vi "test Basic Splitting of Elements.vi"(8 "error in (no error)":errorcluster, 11 "TestCase in":refnum<class "Package List Tests.lvclass">) -> (0 "error out":errorcluster, 3 "TestCase out":refnum<class "Package List Tests.lvclass">)   [LabVIEW 2015, in "Package List Tests.lvclass"]
uses:
  Package List Tests.lvclass
  <vilib>/addons/_JKI Toolkits/VI Tester/TestCase.llb/TestCase.lvclass
  G CLI VIP.lvlib
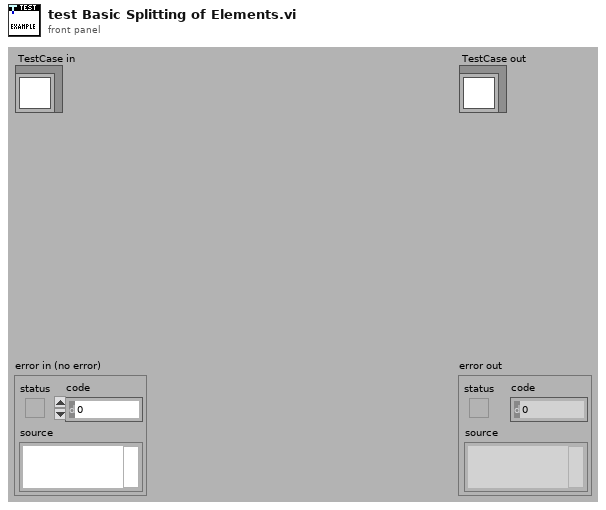
[diagram p1: front panel]
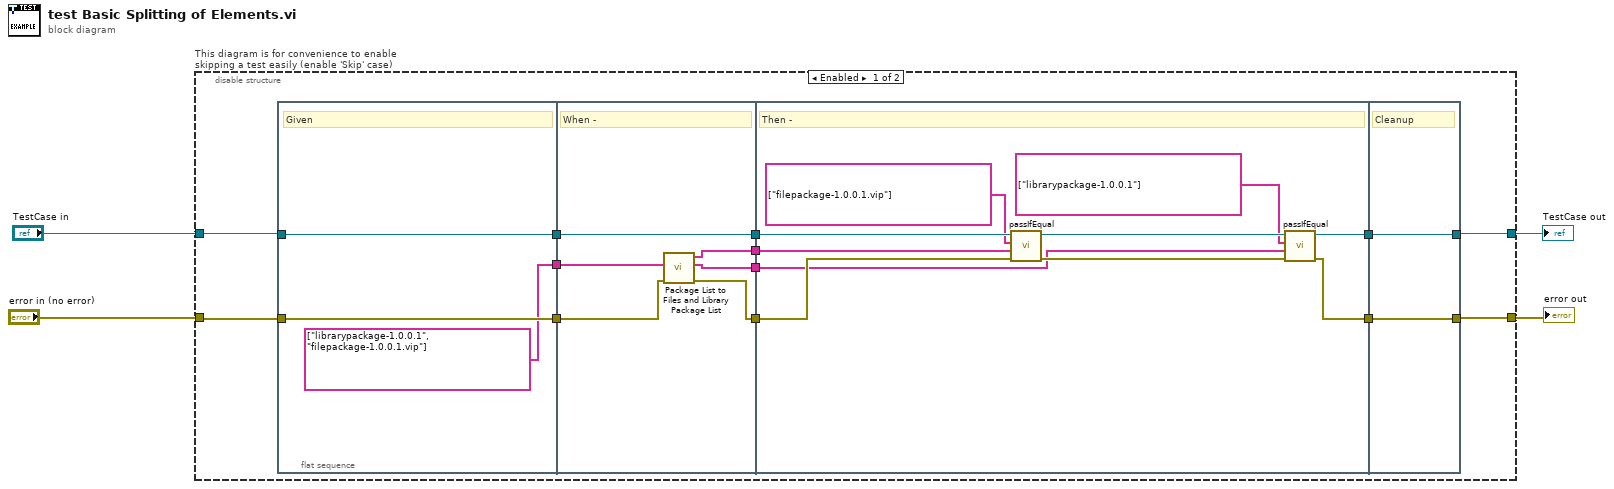
[diagram p0: block diagram]
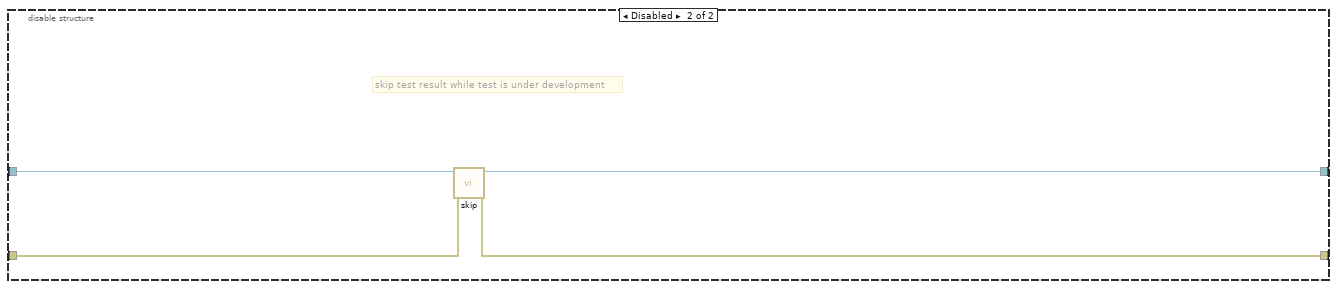
[diagram p2: hidden frame]
diagram:
  n1 = disable-structure "This diagram is for convenience to enable skipping a test easily (enable 'Skip' case)" shown="Enabled" {
    disable-tunnel: "TestCase in" -> [w12 w42]
    disable-tunnel: [w10 w40] -> w1
    disable-tunnel: [w9 w41] -> w3
    disable-tunnel: "error in (no error)" -> [w11 w39]
    frame Enabled {
      n2 = flat-sequence {
        tunnel: w11 -> [w19]
        tunnel: w12 -> [w20]
        tunnel: [w20] -> w17
        tunnel: [w19] -> w16
        tunnel: [string[] ["librarypackage-1.0.0.1", "filepackage-1.0.0.1.vip"]] -> w8
        tunnel: [w26] -> w15
        tunnel: w17 -> [w26]
        tunnel: w16 -> [w22]
        tunnel: w8 -> [w25]
        tunnel: [w24] -> w7
        tunnel: [w23] -> w6
        tunnel: [w21] -> w5
        tunnel: [w31] -> w14
        tunnel: [w32] -> w13
        tunnel: w15 -> [w36]
        tunnel: w7 -> [w30]
        tunnel: w6 -> [w29]
        tunnel: w5 -> [w35]
        tunnel: [w38] -> w9
        tunnel: [w37] -> w10
        tunnel: w14 -> [w37]
        tunnel: w13 -> [w38]
        frame #0 {
          # "Given"
        }
        frame #1 {
          # "When -"
          n3 = call "Package List to Files and Library Package List.vi"("error in (no error)"=w22, "Packages"=w25) -> ("error out"=w21:errorcluster, "Library Packages"=w23:string[], "File Packages"=w24:string[])  [unwired: 7 in]
        }
        frame #2 {
          # "Then -"
          n4 = call-dynamic "passIfEqual.vi"("error in (no error)"=w35, "y"=w30, "x"=string[] ["filepackage-1.0.0.1.vip"], "TestCase in"=w36) -> ("error out"=w33:errorcluster, "TestCase out"=w34:refnum<class "Package List Tests.lvclass">)  [unwired: 6 in]
          n5 = call-dynamic "passIfEqual.vi"("error in (no error)"=w33, "y"=w29, "x"=string[] ["librarypackage-1.0.0.1"], "TestCase in"=w34) -> ("error out"=w32:errorcluster, "TestCase out"=w31:refnum<class "Package List Tests.lvclass">)  [unwired: 6 in]
        }
        frame #3 {
          # "Cleanup"
        }
      }
    }
    frame Disabled {
      # "skip test result while test is under development"
      n6 = call <vilib>:"skip.vi"("error in (no error)"=w39, "TestCase in"=w42) -> ("error out"=w41:errorcluster, "TestCase out"=w40:refnum<class "Package List Tests.lvclass">)  [unwired: 8 in]
    }
  }
  "error out" <- w3
  "TestCase out" <- w1
